vi "Markers.vi"(2 "plot bounds":T1, 3 "Array":string[](array[string])) -> (0 "TextCoords":cluster{"x":i16, "y":i16}[](array[cluster]), 1 "Picture":picture)   [LabVIEW 2020]
doc: "Draw a picture with text inside. Intended use is for (re)labeling tick mark text on y-axis to identify chan displayed at this baseline position.\n\nIt works by looking at the plot area of the graph for which y-axis ticks are to be relabeled, placing text at corresponding vertical positions."
uses:
  <vilib>/Utility/miscctls.llb/LVRectTypeDef.ctl
panel:
  in  "Intan Streaming Data Chart":dbl[][](graph)
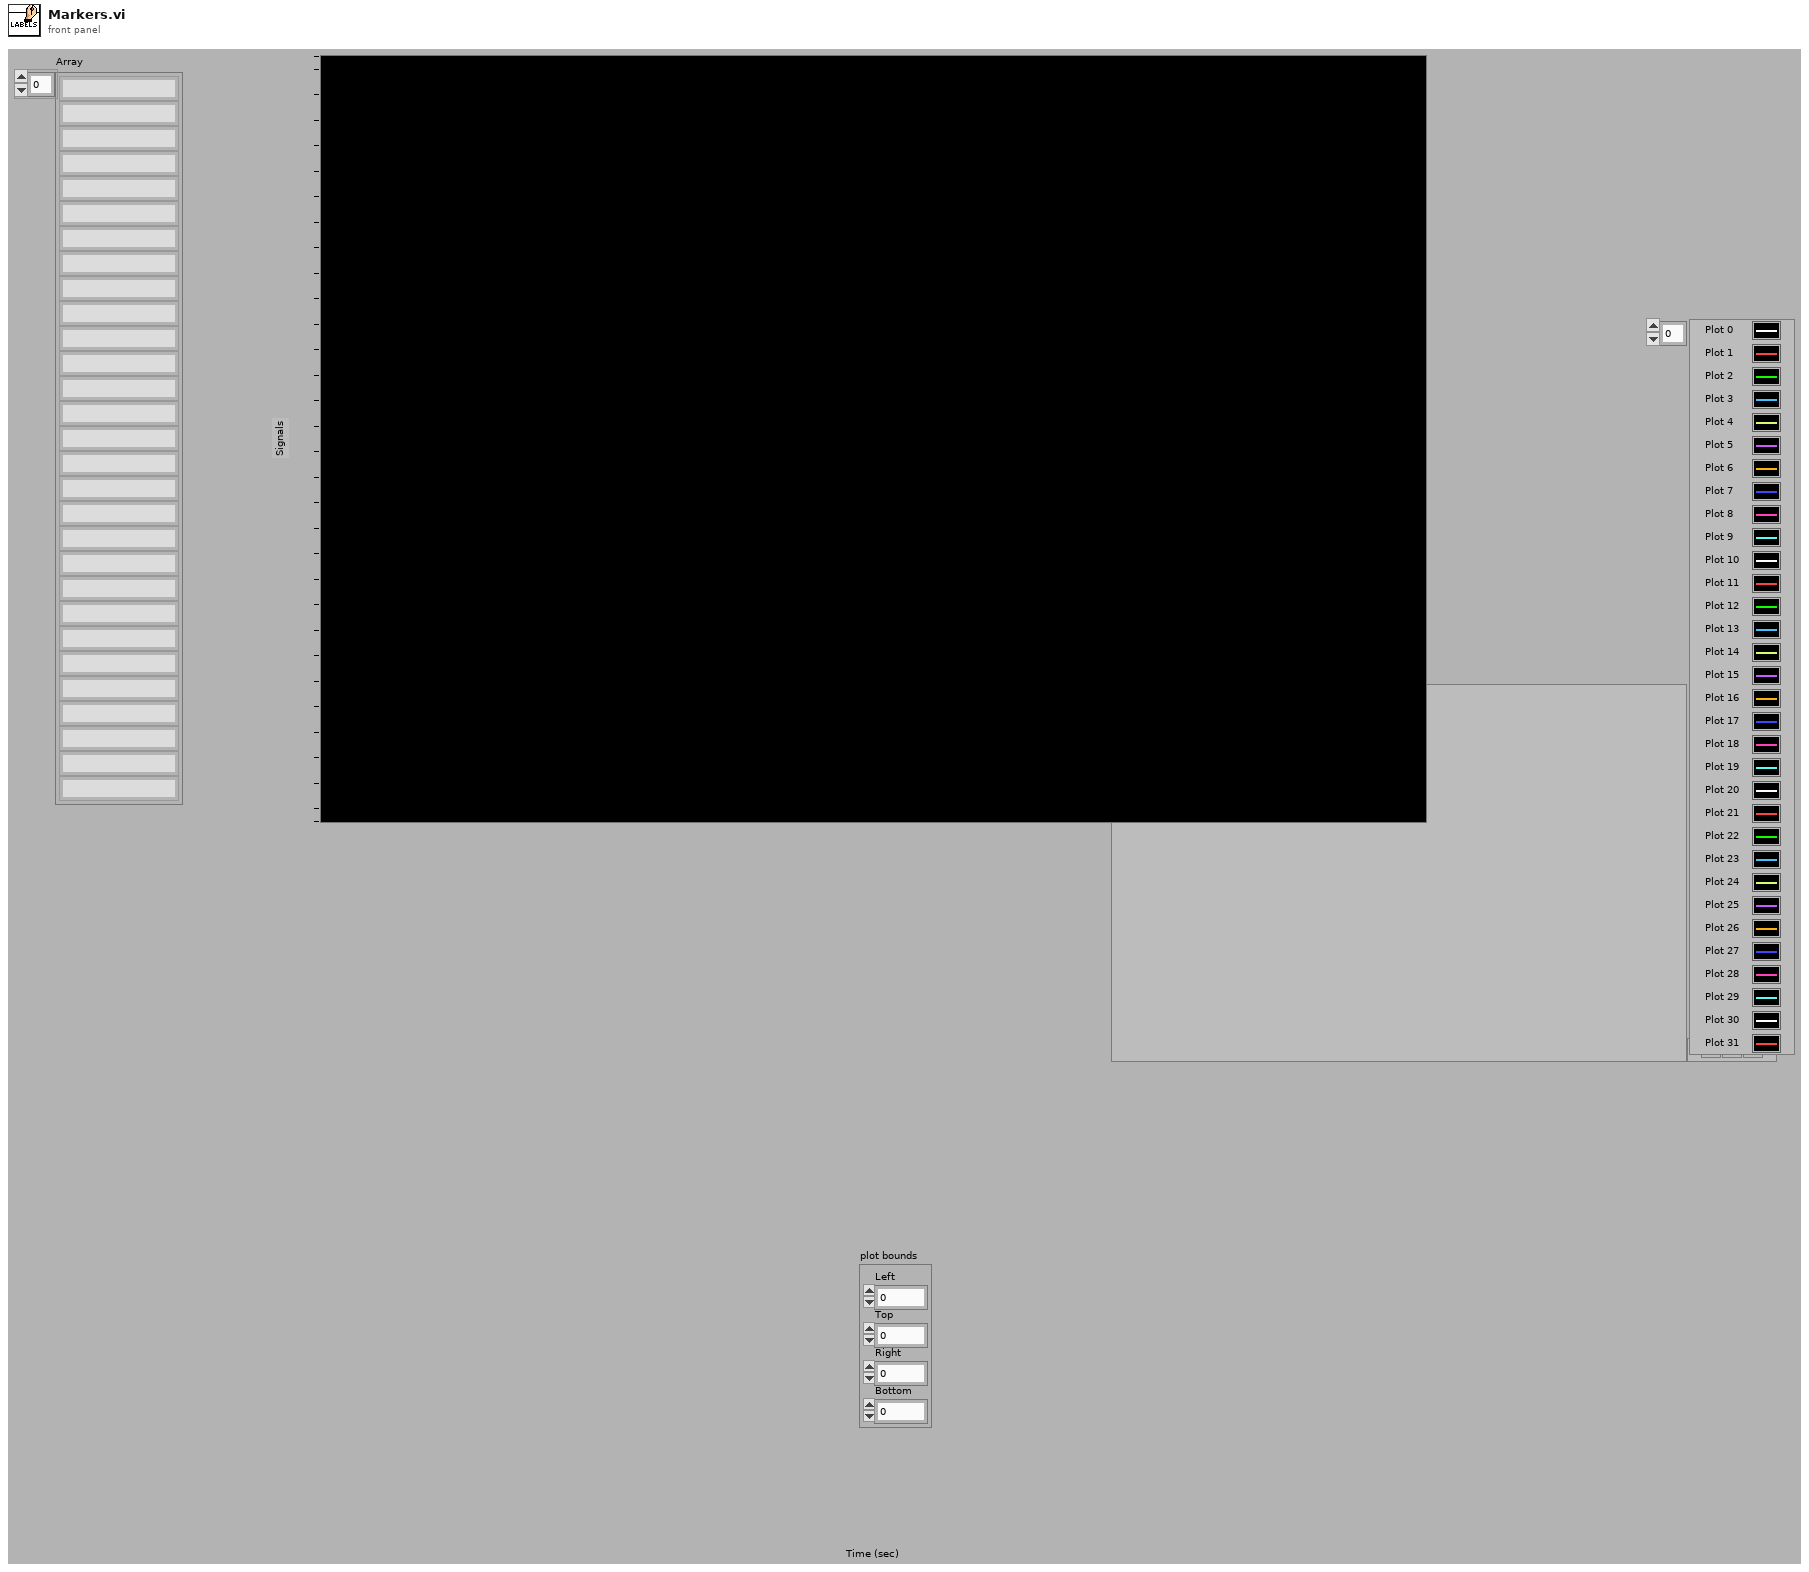
[diagram p1: front panel]
types:
  T1 = typedef "LVRectTypeDef.ctl" = cluster{"Left":i16, "Top":i16, "Right":i16, "Bottom":i16}
  T2 = enum16{"None", "Stacked", "Clockwise", "Counterclockwise"}
  T3 = cluster{"left":i16, "top":i16, "right":i16, "bottom":i16}
  T4 = typedef "LVBoundsTypeDef.ctl" = cluster{"Width":u32, "Height":u32}
  T5 = cluster{"horizontal":enum16{"left", "center", "right"}, "vertical":enum16{"top", "center", "bottom"}}
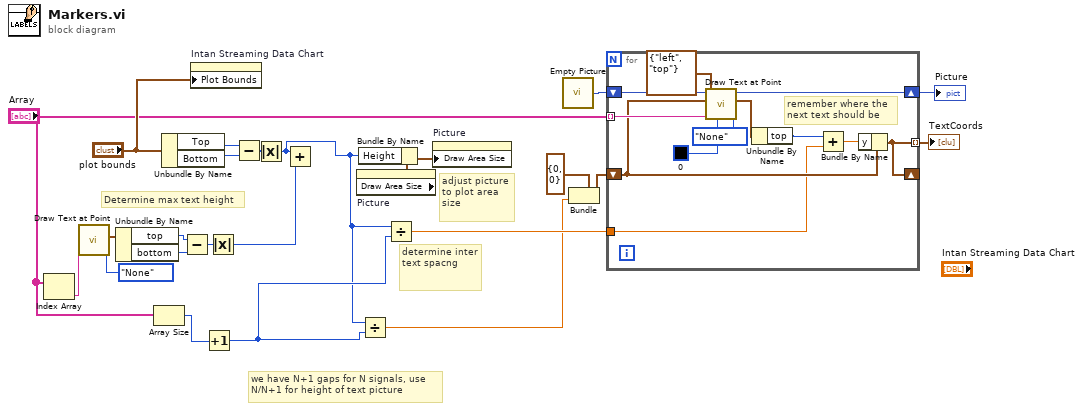
[diagram p0: block diagram]
diagram:
  # "we have N+1 gaps for N signals, use\nN/N+1 for height of text picture"
  # "Determine max text height"
  # "adjust picture to plot area size"
  # "determine inter text spacng"
  n1 = Index Array(array="Array") -> (element=w2:string)  [unwired: 1 in]
  n2 = call <vilib>:"Draw Text at Point.vi"("text orientation"=T2."None", "text"=w2) -> ("text rect"=w7:T3)  [unwired: 8 in, 1 out]
  n3 = Unbundle By Name(w7) -> ("top"=w5:i16, "bottom"=w4:i16)
  n4 = Array Size(array="Array") -> (size(s)=w14:i32)
  n5 = Unbundle By Name("plot bounds") -> ("Top"=w18:i16, "Bottom"=w23:i16)
  n6 = Subtract(x=w5, y=w4) -> (x-y=w3:i16)
  n7 = property on="Intan Streaming Data Chart" class="WFChart (strict)"("Plot Bounds"="plot bounds") -> ()  [unwired: 2 in, 2 out]
  n8 = Increment(x=w14) -> (x+1=w10:i32)
  n9 = Absolute Value(x=w3) -> (abs(x)=w1:i16)
  n10 = Subtract(x=w18, y=w23) -> (x-y=w20:i16)
  n11 = Absolute Value(x=w20) -> (abs(x)=w9:i16)
  n12 = Add(x=w9, y=w1) -> ()  [unwired: 1 out]
  n13 = property on="Picture" class="Pict"() -> ("Draw Area Size"=w22:T4)  [unwired: 2 in, 2 out]
  n14 = Bundle By Name(cluster=w22, "Height"=w9) -> (w21:T4)
  n15 = Divide(x=w9, y=w10) -> (x/y=w11:dbl)
  n16 = Divide(x=w9, y=w10) -> (x/y=w17:dbl)
  n17 = property on="Picture" class="Pict"("Draw Area Size"=w21) -> ()  [unwired: 2 in, 2 out]
  n18 = call "Empty Picture"() -> ("empty picture"=w19:picture)
  n19 = Bundle(cluster=cluster{"x":i16, "y":i16} {"x"=0, "y"=0} ("origin"), "y"=w11) -> (w13:cluster{"x":i16, "y":i16})  [unwired: 1 in]
  n20 = for {
    tunnel: "Array" -> [w34] mode=indexing
    shift-right: [w35] -> w24
    shift-left: w19 -> [w36]
    shift-right: [w26] -> _
    shift-left: w13 -> [w31]
    tunnel: w17 -> [w25]
    tunnel: [w26] -> w16 mode=indexing
    # "remember where the next text should be"
    n21 = call <vilib>:"Draw Text at Point.vi"("text orientation"=T2."None", "text color(black)"=u32 0, "text"=w34, "alignment(left, top)"=T5 {"horizontal"=enum."left", "vertical"=enum."top"}, "origin"=w31, "picture"=w36) -> ("text rect"=w33:T3, "new picture"=w35:picture)  [unwired: 4 in]
    n22 = Unbundle By Name(w33) -> ("top"=w30:i16)
    n23 = Add(x=w30, y=w25) -> (x+y=w29:dbl)
    n24 = Bundle By Name(cluster=w31, "y"=w29) -> (w26:cluster{"x":i16, "y":i16})
  }
  "Picture" <- w24
  "TextCoords" <- w16
